vi "Query Client Connection Status.vi"(8 "error in":errorcluster {"code" format="Error %.0f"}, 11 "NATS Client in":refnum<class "NATS Client.lvclass">) -> (0 "error out":errorcluster {"code" format="Error %.0f"}, 2 "Connected":bool)   [LabVIEW 2024, in "NATS Client.lvlib" / "NATS Client.lvclass"]
doc: "Checks if the Client is connected to the NATS server."
uses:
  NATS Client.lvclass
  NATS Client.lvclass/NATS Client.ctl
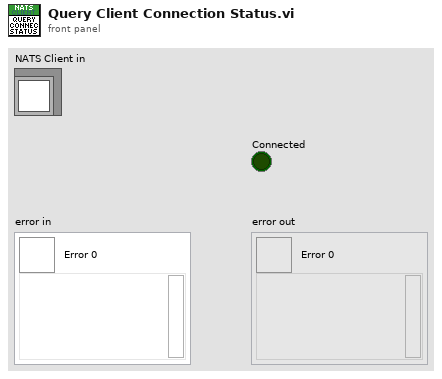
[diagram p1: front panel]
types:
  T1 = typedef "NATS Core.lvlib/nats connection.ctl" = cluster{"connection ID":refnum<k5>, "server INFO":string, "timeout ms":i32, "verbose?":bool, "server headers?":bool, "client headers?":bool}
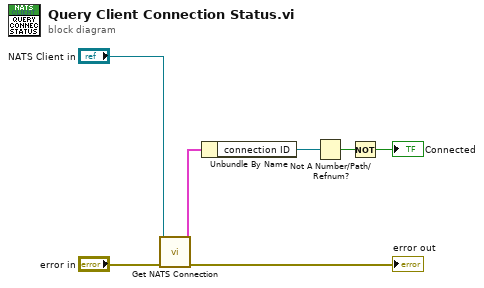
[diagram p0: block diagram]
diagram:
  n1 = call "Get NATS Connection.vi"("error in"="error in", "NATS Client.lvlib:NATS Client.lvclass"="NATS Client in") -> ("error out"=→"error out":errorcluster, "NATS Connection"=w5:T1)  [unwired: 8 in]
  n2 = Unbundle By Name(w5) -> ("connection ID"=w4:refnum<k5>)
  n3 = Not A Number/Path/Refnum?(number/path/refnum=w4) -> (NaN/Path/Refnum?=w3:bool)
  n4 = Not(x=w3) -> (.not. x?=→"Connected":bool)
